vi "RPC_Demo_Template.vi"() -> ()   [LabVIEW 2014]
panel:
  out "Read AValue":dbl
  out "TSMaster Proj List":string(combo)
  # "使用方法：\n1.创建l临时使用的TSMaster 工程\n2.在TSMaster 工程中创建Var0 系统变量\n3.运行此demo \n4.读写Var0  系统变量值"
  # "usage method:\n1. Create a TSMaster project for temporary use\n2. Create Var0 system variables in TSMaster project\n3. Run this demo\n4. Read and write Var0 system variable values"
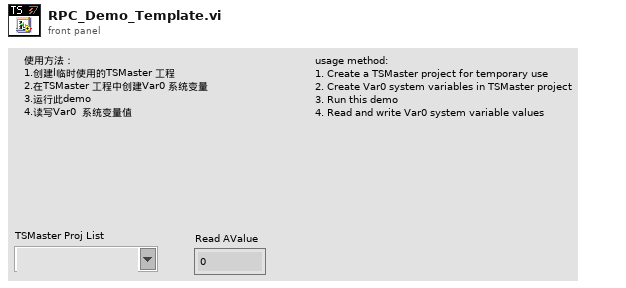
[diagram p1: front panel]
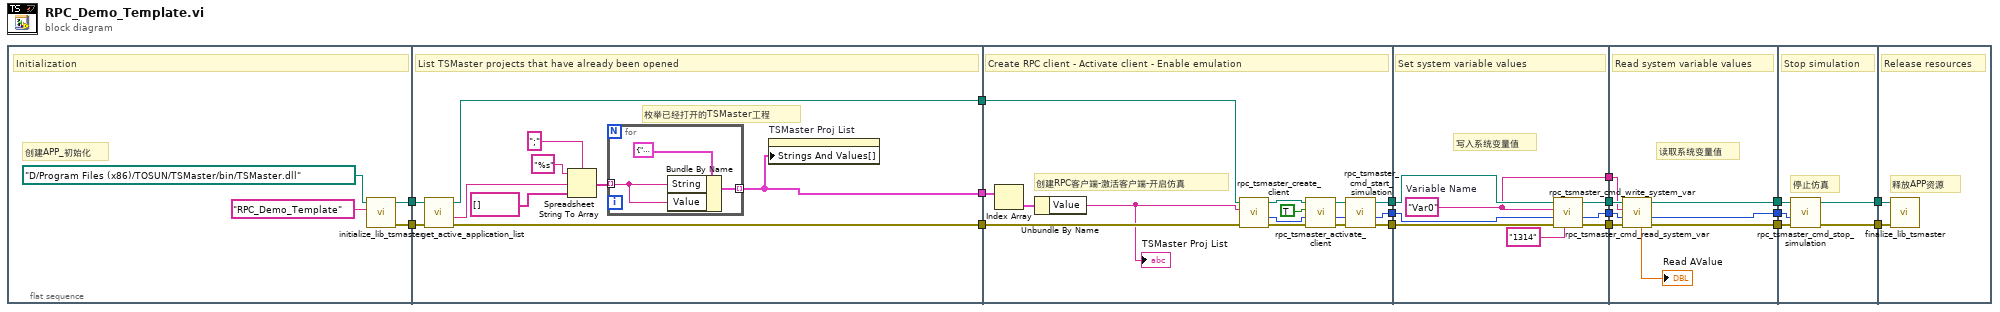
[diagram p0: block diagram]
diagram:
  n1 = flat-sequence {
    tunnel: [w19] -> w17
    tunnel: [w18] -> w16
    tunnel: w17 -> [w28]
    tunnel: w16 -> [w27]
    tunnel: [w24] -> w15
    tunnel: [w23] -> w14
    tunnel: [w22] -> w13
    tunnel: w15 -> [w44]
    tunnel: w14 -> [w43]
    tunnel: w13 -> [w40]
    tunnel: [w38] -> w12
    tunnel: [w37] -> w11
    tunnel: [w36] -> w10
    tunnel: w12 -> [w57]
    tunnel: w11 -> [w56]
    tunnel: w10 -> [w52]
    tunnel: [w54] -> w9
    tunnel: [w53] -> w8
    tunnel: [w51] -> w7
    tunnel: [w50] -> w6
    tunnel: w9 -> [w65]
    tunnel: w8 -> [w64]
    tunnel: w7 -> [w63]
    tunnel: w6 -> [w62]
    tunnel: [w60] -> w5
    tunnel: [w59] -> w4
    tunnel: [w58] -> w3
    tunnel: w5 -> [w70]
    tunnel: w4 -> [w69]
    tunnel: w3 -> [w68]
    tunnel: [w67] -> w2
    tunnel: [w66] -> w1
    tunnel: w2 -> [w72]
    tunnel: w1 -> [w71]
    frame #0 {
      # "创建APP_初始化"
      # "Initialization"
      n2 = call "initialize_lib_tsmaster.vi"("AppName"="RPC_Demo_Template", "Path input"=path "D:/Program Files (x86)/TOSUN/TSMaster/bin/TSMaster.dll") -> ("error output"=w18:errorcluster, "Path output"=w19:path)  [unwired: 8 in]
    }
    frame #1 {
      # "枚举已经打开的TSMaster工程"
      # "List TSMaster projects that have already been opened"
      n3 = call "get_active_application_list.vi"("error in"=w27, "path in"=w28) -> ("error out"=w23:errorcluster, "ATSMasterAppNames"=w26:string, "path out"=w24:path)  [unwired: 6 in, 1 out]
      n4 = Spreadsheet String To Array(delimiter (Tab)=";" ("分隔符(Tab)"), format string="%s", spreadsheet string=w26, array type (2D Dbl)=string[] []) -> (array=w25:string[])
      n5 = for {
        tunnel: w25 -> [w33] mode=indexing
        tunnel: [w32] -> w22 mode=indexing
        n6 = Bundle By Name(cluster=cluster{"String":string, "Value":string} {"String"="", "Value"=""}, "String"=w33, "Value"=w33) -> (w32:cluster{"String":string, "Value":string})
      }
      n7 = property on="TSMaster Proj List" class="CmbBox"("Strings And Values[]"=w22) -> ()  [unwired: 2 in, 2 out]
    }
    frame #2 {
      # "创建RPC客户端-激活客户端-开启仿真"
      # "Create RPC client - Activate client - Enable emulation"
      n8 = Index Array(array=w40) -> (element=w39:cluster{"String":string, "Value":string})  [unwired: 1 in]
      n9 = Unbundle By Name(w39) -> ("Value"=w35:string)
      "TSMaster Proj List" <- w35
      n10 = call "rpc_tsmaster_create_client.vi"("error in (no error)"=w43, "AppName"=w35, "Path input"=w44) -> ("error output"=w41:errorcluster, "AHandle"=w46:i32, "Path output"=w49:path)  [unwired: 5 in, 1 out]
      n11 = call "rpc_tsmaster_activate_client.vi"("error in (no error)"=w41, "AHandle"=w46, "AActivate"=TRUE, "Path input"=w49) -> ("error output"=w47:errorcluster, "AHandle 2"=w45:i32, "Path output"=w48:path)  [unwired: 4 in, 1 out]
      n12 = call "rpc_tsmaster_cmd_start_simulation.vi"("error in (no error)"=w47, "AHandle"=w45, "路径输入"=w48) -> ("error out"=w37:errorcluster, "AHandle 2"=w36:u32, "路径输出"=w38:path)  [unwired: 5 in, 1 out]
    }
    frame #3 {
      w51 = "Var0"  # Variable Name
      # "写入系统变量值"
      # "Set system variable values"
      n13 = call "rpc_tsmaster_cmd_write_system_var.vi"("AValue"="1314", "error in (no error)"=w56, "AHandle"=w52, "ACompleteName"=w51, "Path input"=w57) -> ("error output"=w53:errorcluster, "AHandle out"=w50:i32, "Path output"=w54:path)  [unwired: 3 in, 1 out]
    }
    frame #4 {
      # "读取系统变量值"
      # "Read system variable values"
      n14 = call "rpc_tsmaster_cmd_read_system_var.vi"("error in (no error)"=w64, "AHandle"=w62, "ASysVarName"=w63, "Path input"=w65) -> ("error output"=w59:errorcluster, "AHandle out"=w58:u32, "Path output"=w60:path, "AValue"=→"Read AValue":dbl)  [unwired: 3 in, 1 out]
    }
    frame #5 {
      # "停止仿真"
      # "Stop simulation"
      n15 = call "rpc_tsmaster_cmd_stop_simulation.vi"("error in (no error)"=w69, "AHandle"=w68, "路径输入"=w70) -> ("error out"=w66:errorcluster, "路径输出"=w67:path)  [unwired: 6 in, 1 out]
    }
    frame #6 {
      # "释放APP资源"
      # "Release resources"
      n16 = call "finalize_lib_tsmaster.vi"("error in (no error)"=w71, "Path"=w72) -> ()  [unwired: 8 in, 2 out]
    }
  }
